vi "CreateFolder.vi"(8 "error in":errorcluster, 11 "folder":path) -> (0 "error out":errorcluster, 3 "folder out":path)   [LabVIEW 2017, in "TraceLogger.lvlib"]
uses:
  <vilib>/addons/TraceLogger/TraceLogger.lvlib
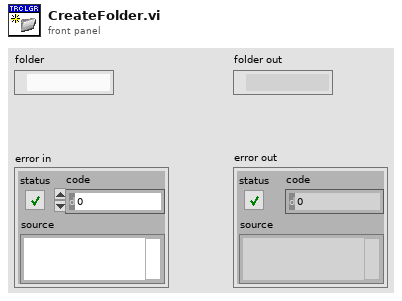
[diagram p1: front panel]
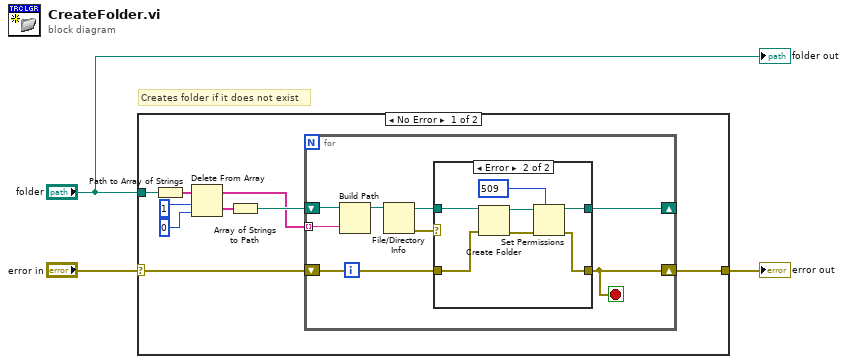
[diagram p0: block diagram]
diagram:
  # "Creates folder if it does not exist"
  n1 = case shown="No Error" "error in" {
    selector: "error in" -> [w5 w30]
    tunnel: [w12 w30] -> w2
    tunnel: "folder" -> [w4 _]
    frame No Error {
      n2 = Path to Array of Strings(0:w4) -> (2:w11:string[])  [unwired: 1 out]
      n3 = Delete From Array(array=w11, length=1, index=0) -> (deleted portion=w8:string[], array with subset deleted=w6:string[])
      n4 = Array of Strings to Path(0:w8) -> (2:w10:path)  [unwired: 1 out]
      n5 = for {
        shift-right: [w16] -> _
        shift-left: w10 -> [w20]
        tunnel: w6 -> [w19] mode=indexing
        shift-right: [w13] -> w12
        shift-left: w5 -> [w15]
        stop <- w13 stop-if-true
        n6 = Build Path(base path=w20, name or relative path=w19) -> (appended path=w18:path)
        n7 = File/Directory Info(path=w18) -> (path out=w17:path, error out=w14:errorcluster)  [unwired: 1 in, 5 out]
        n8 = case shown="Error" w14 {
          tunnel: [w22 w24] -> w16
          tunnel: w17 -> [w22 w28]
          tunnel: w15 -> [w21 w29]
          tunnel: [w21 w23] -> w13
          frame No Error {
          }
          frame Error {
            n9 = Create Folder(path (use dialog)=w28, error in=w29) -> (created path=w26:path, error out=w25:errorcluster)  [unwired: 2 out]
            n10 = Set Permissions(7:i16 509 ("permissions"), 8:w25, 11:w26) -> (0:w23:errorcluster, 3:w24:path)  [unwired: 2 in]
          }
        }
      }
    }
    frame Error {
    }
  }
  "error out" <- w2
  "folder out" <- "folder"
